vi "CheckColision.vi"(8 "error in (no error)":errorcluster, 10 "Clicked Square":map{string, i32}(c390), 11 "object in":refnum<class "Board.lvclass">) -> (0 "error out":errorcluster, 3 "object out":refnum<class "Board.lvclass">)   [LabVIEW 2020, in "Board.lvclass"]
doc: "Checks if the selected piece will colide with another piece and, if so and piece same color, remove all squares from pattern at the colision spot and further. If oposit color, keep the colition square but delete further elements"
uses:
  Board.lvclass
  Pieces/Piece.lvclass
panel:
  out "Array":map{string, i32}[](array[numeric])
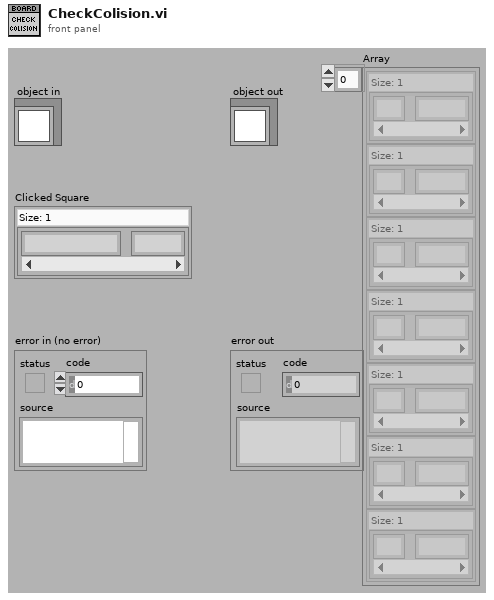
[diagram p1: front panel]
types:
  T1 = typedef "Board.lvclass/pieceMap.ctl" = map{map{string, i32}, refnum<class "Piece.lvclass">}
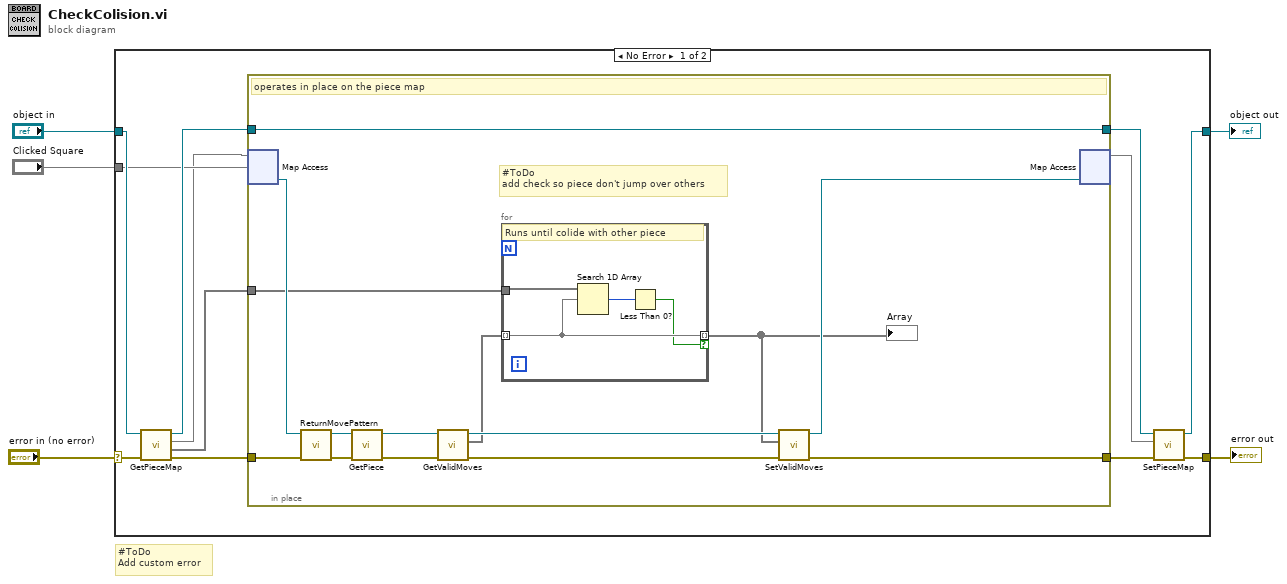
[diagram p0: block diagram]
diagram:
  # "#ToDo\nAdd custom error"
  n1 = case shown="No Error" "error in (no error)" {
    selector: "error in (no error)" -> [w9 w37]
    tunnel: [w12 w37] -> w5
    tunnel: [w10 w36] -> w3
    tunnel: "object in" -> [w11 w36]
    tunnel: "Clicked Square" -> [w8 _]
    frame No Error {
      n2 = call "GetPieceMap.vi"("error in (no error)"=w9, "object in"=w11) -> ("error out"=w16:errorcluster, "All Pieces"=w7:map{string, i32}[], "pieceMap"=w6:T1, "object out"=w14:refnum<class "Board.lvclass">)  [unwired: 6 in]
      n3 = in-place {
        in-place-border: w16 -> [w30]
        in-place-border: [w26] -> w15
        in-place-border: w14 -> [w29]
        in-place-border: [w29] -> w13
        in-place-border: w7 -> [w18]
        # "#ToDo\nadd check so piece don't jump over others"
        # "operates in place on the piece map"
        n4 = in-place-map #1(w6, w8) -> (w31:refnum<class "Piece.lvclass">)  [unwired: 1 in, 1 out]
        n5 = call-dynamic "ReturnMovePattern.vi"("error in (no error)"=w30, "object in"=w31) -> ("error out"=w27:errorcluster, "object out"=w22:refnum<class "Piece.lvclass">)  [unwired: 8 in]
        n6 = call "GetPiece.vi"("error in (no error)"=w27, "Piece in"=w22) -> ("error out"=w23:errorcluster, "Piece out"=w21:refnum<class "Piece.lvclass">)  [unwired: 5 in, 3 out]
        n7 = call "GetValidMoves.vi"("error in (no error)"=w23, "object in"=w21) -> ("error out"=w28:errorcluster, "validMoves"=w20:map{string, i32}[], "object out"=w25:refnum<class "Piece.lvclass">)  [unwired: 7 in]
        n8 = for {
          tunnel: w20 -> [w34] mode=indexing
          tunnel: [w34] -> w19 mode=indexing if=w32
          tunnel: w18 -> [w35]
          # "Runs until colide with other piece"
          n9 = Search 1D Array(1D array=w35, element=w34) -> (index of element=w33:i32)  [unwired: 1 in]
          n10 = Less Than 0?(x=w33) -> (x < 0?=w32:bool)
        }
        "Array" <- w19
        n11 = call "SetValidMoves.vi"("error in (no error)"=w28, "validMoves"=w19, "object in"=w25) -> ("error out"=w26:errorcluster, "object out"=w24:refnum<class "Piece.lvclass">)  [unwired: 7 in]
        n12 = in-place-map #1(w24) -> (w17:T1)  [unwired: 1 in, 2 out]
      }
      n13 = call "SetPieceMap.vi"("error in (no error)"=w15, "pieceMap"=w17, "object in"=w13) -> ("error out"=w12:errorcluster, "object out"=w10:refnum<class "Board.lvclass">)  [unwired: 7 in]
    }
    frame Error {
    }
  }
  "error out" <- w5
  "object out" <- w3
